vi "sub vi - cycle&temp fail v2.vi"(0 "Amps Lo?":bool, 2 "Input Cluster":T1, 3 "SELECT":T2(ring), 4 "Amps Hi?":bool) -> (15 "(FAIL) out":cluster{"FAIL LO":dbl, "FAIL HI":dbl}, 16 "(DISP) out":T3, 17 "(RESULT) out":bool, 19 "file error":errorcluster)   [LabVIEW 2013]
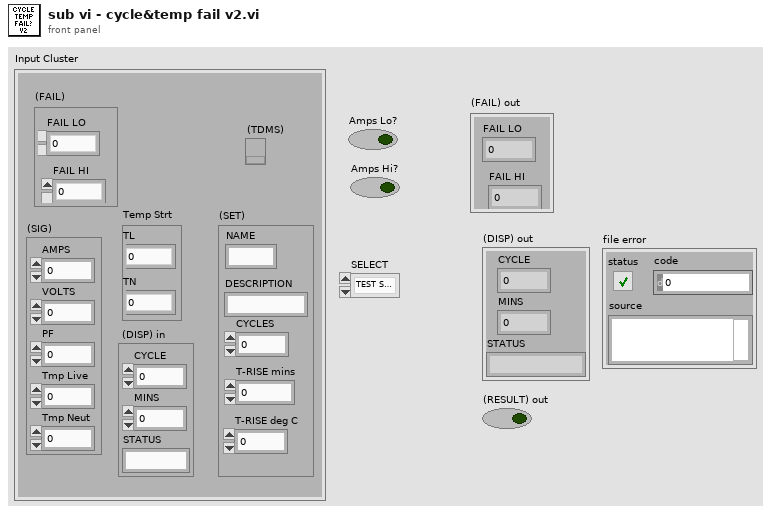
[diagram p1: front panel]
types:
  T1 = cluster{"(FAIL)":cluster{"FAIL LO":dbl, "FAIL HI":dbl}, "(SIG)":cluster{"AMPS":dbl, "VOLTS":dbl, "PF":dbl, "Tmp Live":dbl, "Tmp Neut":dbl}, "Temp Strt":cluster{"TL":dbl, "TN":dbl}, " (DISP) in":cluster{"CYCLE":dbl, "MINS":dbl, "STATUS":string}, "(SET)":cluster{"NAME":string, "DESCRIPTION":string, "CYCLES":dbl, "T-RISE mins":dbl, "T-RISE deg C":dbl}, "(TDMS)":refnum<k34>}
  T2 = enum32{"TEST SET UP", "CYCLE TEST", "T-RISE TEST"}
  T3 = cluster{"CYCLE":dbl, "MINS":dbl, "STATUS":string}
  T4 = cluster{"AMPS":dbl, "VOLTS":dbl, "PF":dbl, "Tmp Live":dbl, "Tmp Neut":dbl}
  T5 = cluster{"NAME":string, "DESCRIPTION":string, "CYCLES":dbl, "T-RISE mins":dbl, "T-RISE deg C":dbl}
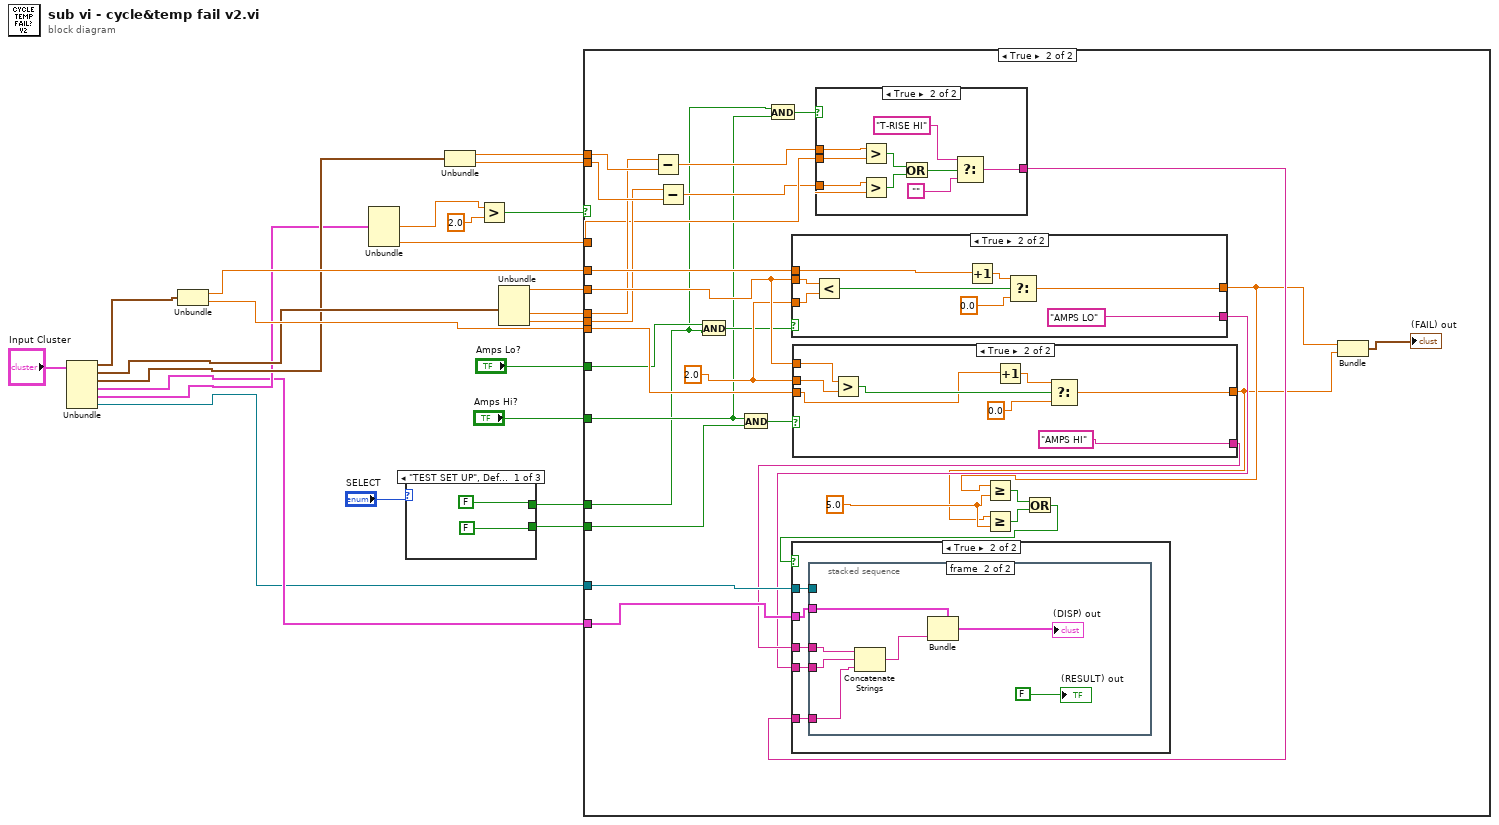
[diagram p0: block diagram]
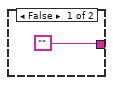
[diagram p3: hidden frame]
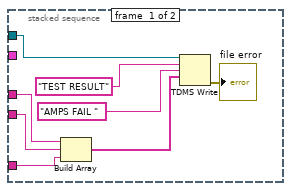
[diagram p5: hidden frame]
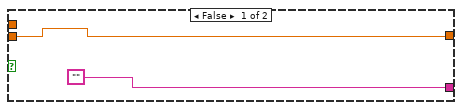
[diagram p6: hidden frame]
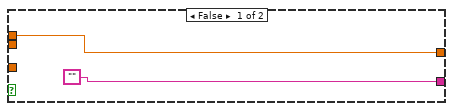
[diagram p7: hidden frame]
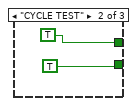
[diagram p8: hidden frame]
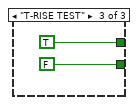
[diagram p9: hidden frame]
diagram:
  n1 = Unbundle("Input Cluster") -> ("(FAIL)"=w8:cluster{"FAIL LO":dbl, "FAIL HI":dbl}, "(SIG)"=w5:T4, "Temp Strt"=w4:cluster{"TL":dbl, "TN":dbl}, "(DISP) in"=w2:T3, "(SET)"=w3:T5, "(TDMS)"=w1:refnum<k34>)
  n2 = Unbundle(w8) -> ("FAIL LO"=w7:dbl, "FAIL HI"=w6:dbl)
  n3 = Unbundle(w3) -> ("CYCLES"=w12:dbl, "T-RISE deg C"=w17:dbl)  [unwired: 3 out]
  n4 = case shown="\"TEST SET UP\", Default" "SELECT" {
    tunnel: [FALSE TRUE TRUE] -> w13
    tunnel: [FALSE TRUE FALSE] -> w16
    frame "TEST SET UP", Default {
    }
    frame "CYCLE TEST" {
    }
    frame "T-RISE TEST" {
    }
  }
  n5 = Unbundle(w4) -> ("TL"=w21:dbl, "TN"=w20:dbl)
  n6 = Greater?(x=w12, y=2.0) -> (0:w10:bool)
  n7 = Unbundle(w5) -> ("AMPS"=w22:dbl, "Tmp Live"=w19:dbl, "Tmp Neut"=w18:dbl)  [unwired: 2 out]
  n8 = case shown="True" w10 {
    tunnel: w22 -> [_ w59]
    tunnel: w7 -> [_ w57]
    tunnel: w6 -> [_ w56]
    tunnel: w1 -> [_ w55]
    tunnel: w2 -> [_ w54]
    tunnel: w21 -> [_ w53]
    tunnel: w20 -> [_ w52]
    tunnel: w19 -> [_ w51]
    tunnel: w18 -> [_ w50]
    tunnel: w17 -> [_ w49]
    tunnel: w16 -> [_ w38]
    tunnel: "Amps Lo?" -> [_ w36]
    tunnel: "Amps Hi?" -> [_ w34]
    tunnel: w13 -> [_ w33]
    frame False {
    }
    frame True {
      w41 = 5.0
      w58 = 2.0
      n9 = Subtract(x=w51, y=w53) -> (x-y=w48:dbl)
      n10 = Subtract(x=w50, y=w52) -> (x-y=w47:dbl)
      n11 = And(x=w36, y=w33) -> (x .and. y?=w37:bool)
      n12 = And(x=w34, y=w38) -> (x .and. y?=w39:bool)
      n13 = And(x=w33, y=w34) -> (x .and. y?=w35:bool)
      n14 = case shown="True" w37 {
        tunnel: w59 -> [_ w109]
        tunnel: ["" "AMPS LO"] -> w45
        tunnel: w58 -> [_ w107]
        tunnel: w57 -> [w100 w103]
        tunnel: [w100 w102] -> w32
        frame False {
        }
        frame True {
          n15 = Less?(x=w109, y=w107) -> (x < y?=w106:bool)
          n16 = Increment(x=w103) -> (x+1=w105:dbl)
          n17 = Select(t=w105, s=w106, f=0.0) -> (s? t:f=w102:dbl)
        }
      }
      n18 = case shown="True" w39 {
        tunnel: w59 -> [_ w99]
        tunnel: ["" "AMPS HI"] -> w46
        tunnel: w58 -> [_ w97]
        tunnel: [w90 w93] -> w31
        tunnel: w56 -> [w90 w92]
        frame False {
        }
        frame True {
          n19 = Greater?(x=w99, y=w97) -> (0:w96:bool)
          n20 = Increment(x=w92) -> (x+1=w95:dbl)
          n21 = Select(t=w95, s=w96, f=0.0) -> (s? t:f=w93:dbl)
        }
      }
      n22 = case shown="True" w35 {
        tunnel: w49 -> [_ w69]
        tunnel: w48 -> [_ w68]
        tunnel: w47 -> [_ w67]
        tunnel: ["" w61] -> w40
        frame False {
        }
        frame True {
          n23 = Greater?(x=w68, y=w69) -> (0:w65:bool)
          n24 = Greater?(x=w67, y=w69) -> (0:w66:bool)
          n25 = Or(x=w65, y=w66) -> (x .or. y?=w62:bool)
          n26 = Select(t="T-RISE HI", s=w62, f="") -> (s? t:f=w61:string)
        }
      }
      n27 = Greater Or Equal?(x=w32, y=w41) -> (x >= y?=w44:bool)
      n28 = Greater Or Equal?(x=w31, y=w41) -> (x >= y?=w43:bool)
      n29 = Or(x=w44, y=w43) -> (x .or. y?=w42:bool)
      n30 = case shown="True" w42 {
        tunnel: w46 -> [_ w74]
        tunnel: w45 -> [_ w73]
        tunnel: w54 -> [_ w72]
        tunnel: w55 -> [_ w71]
        tunnel: w40 -> [_ w70]
        frame False {
        }
        frame True {
          n31 = stacked-sequence {
            tunnel: w74 -> [w81 w89]
            tunnel: w73 -> [w80 w88]
            tunnel: w72 -> [_ w86]
            tunnel: w71 -> [w76 _]
            tunnel: w70 -> [w75 w85]
            frame #0 {
              n32 = Build Array(w81, w80, w75) -> (w79:string[])
              n33 = TDMS Write(0:w76, 5:"TEST RESULT", 7:"AMPS FAIL ", 9:w79) -> (15:→"file error":errorcluster)  [unwired: 2 in, 3 out]
            }
            frame #1 {
              n34 = Concatenate Strings(w89, w88, w85) -> (w87:string)
              n35 = Bundle(cluster=w86, "STATUS"=w87) -> (→"(DISP) out":T3)  [unwired: 2 in]
              "(RESULT) out" <- FALSE
            }
          }
        }
      }
      n36 = Bundle("FAIL LO"=w32, "FAIL HI"=w31) -> (→"(FAIL) out":cluster{"FAIL LO":dbl, "FAIL HI":dbl})  [unwired: 1 in]
    }
  }
